vi "Query Current.vi"(8 "error in (no error)":errorcluster, 11 "Agilent 6xxx in":refnum<class "Agilent 6xxx.lvclass">) -> (0 "error out":errorcluster, 2 "Current":dbl, 3 "Agilent 6xxx out":refnum<class "Agilent 6xxx.lvclass">)   [LabVIEW 2020, in "Agilent 6xxx.lvclass"]
uses:
  Agilent 6xxx.lvclass
  C:/Sandbox/Git_Sandbox/WiSpry Test Framework source code (LV20)/WiSpry Test Framework/Instruments/Instrument.lvclass
  C:/Sandbox/Git_Sandbox/WiSpry Test Framework source code (LV20)/WiSpry Test Framework/Instruments/Power Supply/Power Supply.lvclass
  Power Supply.lvclass/Power Supply.ctl
  Instrument.lvclass/Instrument.ctl
  Power Supply.lvclass
  Instrument.lvclass
  <instrlib>/Agilent 6XXX Series/Agilent 6XXX Series.lvlib
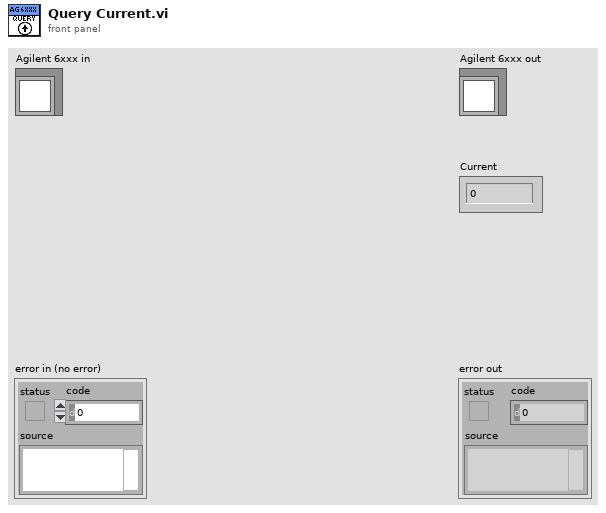
[diagram p1: front panel]
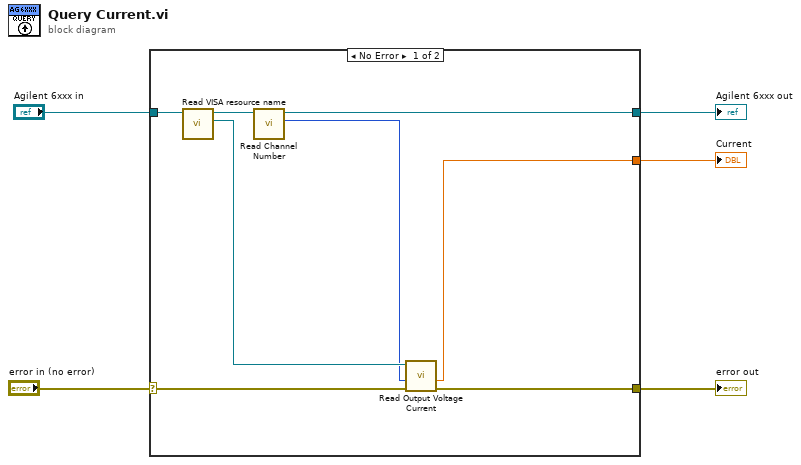
[diagram p0: block diagram]
diagram:
  n1 = case shown="No Error" "error in (no error)" {
    selector: "error in (no error)" -> [w10 w14]
    tunnel: [w11 w15] -> w2
    tunnel: "Agilent 6xxx in" -> [w12 w15]
    tunnel: [w7 w14] -> w4
    tunnel: [w6 _] -> w3
    frame No Error {
      n2 = call "Read VISA resource name.vi"("Instrument in"=w12) -> ("VISA resource name"=w9:refnum<visa-resource-name>, "Instrument out"=w13:refnum<class "Agilent 6xxx.lvclass">)  [unwired: 9 in]
      n3 = call "Read Channel Number.vi"("Power Supply in"=w13) -> ("Channel Number"=w8:u8, "Power Supply out"=w11:refnum<class "Agilent 6xxx.lvclass">)  [unwired: 9 in]
      n4 = call <instrlib>:"Read Output Voltage Current.vi"("error in (no error)"=w10, "channel (1)"=w8, "VISA resource name"=w9) -> ("error out"=w7:errorcluster, "output current"=w6:dbl)  [unwired: 5 in, 2 out]
    }
    frame Error {
    }
  }
  "error out" <- w4
  "Agilent 6xxx out" <- w2
  "Current" <- w3
